vi "LaserPIDPositioning.vi"() -> ()   [LabVIEW 2014]
uses:
  <vilib>/addons/control/pid/pid.llb/PID (DBL).vi
  <vilib>/vision/NI_Vision_Development_Module.lvlib
  <vilib>/addons/control/pid/NI_PID_pid.lvlib
panel:
  out "error out":errorcluster
  in  "error in":errorcluster
  in  "Destination Point":cluster{"DestinationX":dbl, "DestinationY":dbl}
  in  "Horizontal Edge":T1 {"Point2 (Real-World)"."Y" format="%.2f"; "Point2 (Real-World)"."X" format="%.2f"; "Point1 (Real-World)"."Y" format="%.2f"; "Point1 (Real-World)"."X" format="%.2f"; "Point2 (Pixels)"."Y" format="%.2f"; "Point2 (Pixels)"."X" format="%.2f"; "Point1 (Pixels)"."Y" format="%.2f"; "Point1 (Pixels)"."X" format="%.2f"}
  in  "Vertical Edge":T1 {"Point2 (Real-World)"."Y" format="%.2f"; "Point2 (Real-World)"."X" format="%.2f"; "Point1 (Real-World)"."Y" format="%.2f"; "Point1 (Real-World)"."X" format="%.2f"; "Point2 (Pixels)"."Y" format="%.2f"; "Point2 (Pixels)"."X" format="%.2f"; "Point1 (Pixels)"."Y" format="%.2f"; "Point1 (Pixels)"."X" format="%.2f"}
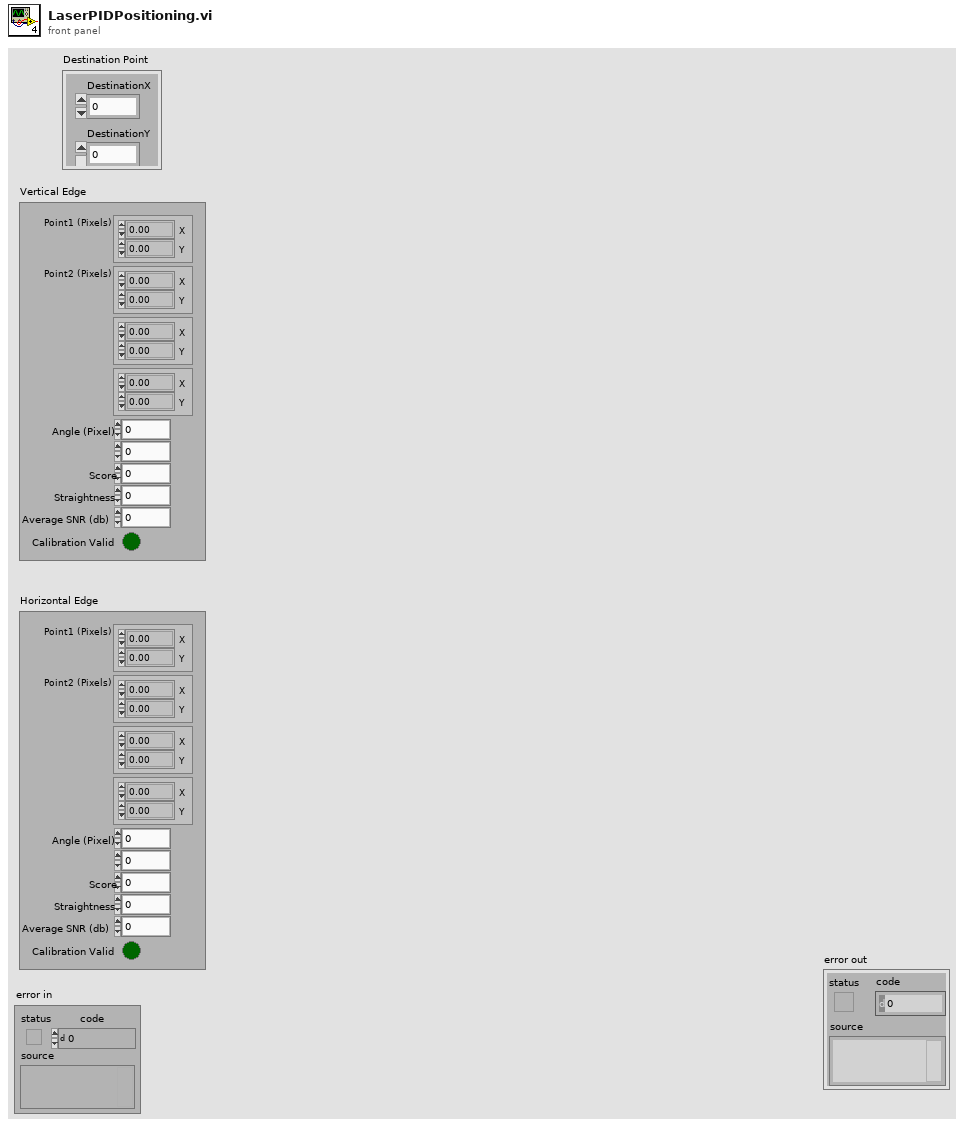
[diagram p1: front panel]
types:
  T1 = cluster{"Point1 (Pixels)":cluster{"X":sgl, "Y":sgl}, "Point2 (Pixels)":cluster{"X":sgl, "Y":sgl}, "Point1 (Real-World)":cluster{"X":sgl, "Y":sgl}, "Point2 (Real-World)":cluster{"X":sgl, "Y":sgl}, "Angle (Pixel)":dbl, "Angle (Real-World)":dbl, "Score":dbl, "Straightness":dbl, "Average SNR (db)":dbl, "Calibration Valid":bool}
  T2 = cluster{"proportional gain (Kc)":dbl, "integral time (Ti, min)":dbl, "derivative time (Td, min)":dbl}
  T3 = cluster{cluster{"X":sgl, "Y":sgl}, cluster{"X":sgl, "Y":sgl}}
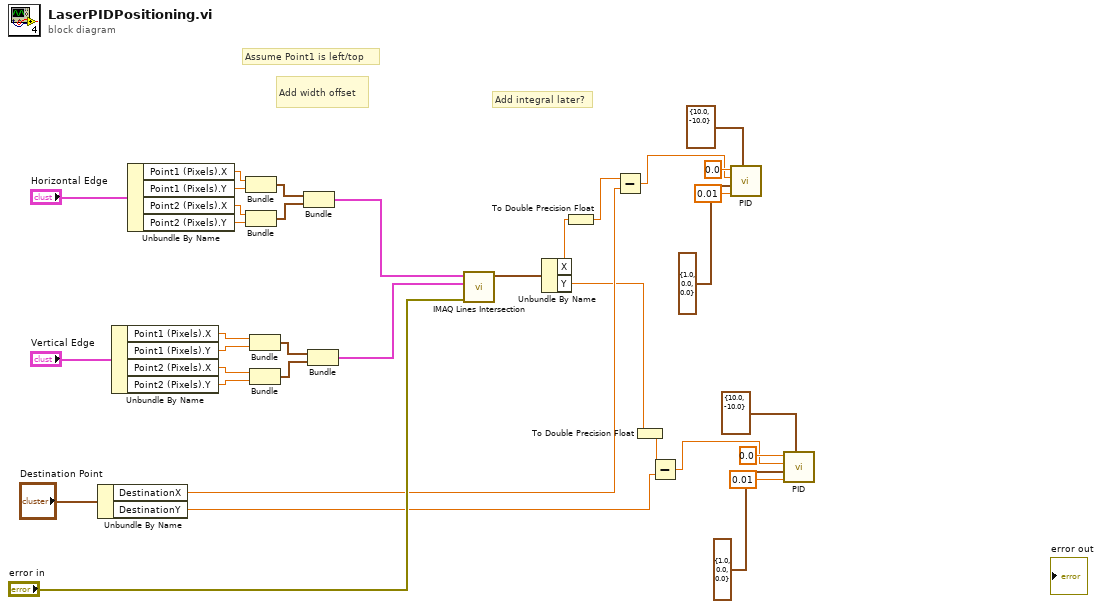
[diagram p0: block diagram]
diagram:
  # "Add integral later?"
  # "Add width offset"
  # "Assume Point1 is left/top"
  n1 = Unbundle By Name("Destination Point") -> ("DestinationX"=w13:dbl, "DestinationY"=w6:dbl)
  n2 = Unbundle By Name("Vertical Edge") -> ("Point1 (Pixels).X"=w23:sgl, "Point1 (Pixels).Y"=w22:sgl, "Point2 (Pixels).X"=w21:sgl, "Point2 (Pixels).Y"=w20:sgl)
  n3 = Unbundle By Name("Horizontal Edge") -> ("Point1 (Pixels).X"=w32:sgl, "Point1 (Pixels).Y"=w31:sgl, "Point2 (Pixels).X"=w30:sgl, "Point2 (Pixels).Y"=w29:sgl)
  n4 = Bundle("X"=w32, "Y"=w31) -> (w28:cluster{"X":sgl, "Y":sgl})  [unwired: 1 in]
  n5 = Bundle("X"=w30, "Y"=w29) -> (w27:cluster{"X":sgl, "Y":sgl})  [unwired: 1 in]
  n6 = Bundle("X"=w23, "Y"=w22) -> (w25:cluster{"X":sgl, "Y":sgl})  [unwired: 1 in]
  n7 = Bundle("X"=w21, "Y"=w20) -> (w24:cluster{"X":sgl, "Y":sgl})  [unwired: 1 in]
  n8 = Bundle(w28, w27) -> (w26:T3)  [unwired: 1 in]
  n9 = Bundle(w25, w24) -> (w19:T3)  [unwired: 1 in]
  n10 = call "IMAQ Lines Intersection"("error in (no error)"="error in", "Line 2"=w19, "Line 1"=w26) -> ("Intersection Point"=w17:cluster{"X":sgl, "Y":sgl})  [unwired: 6 in, 2 out]
  n11 = Unbundle By Name(w17) -> ("X"=w3:sgl, "Y"=w7:sgl)
  n12 = To Double Precision Float(number=w3) -> (double precision float=w2:dbl)
  n13 = Subtract(x=w2, y=w13) -> (x-y=w12:dbl)
  n14 = To Double Precision Float(number=w7) -> (double precision float=w1:dbl)
  n15 = Subtract(x=w1, y=w6) -> (x-y=w8:dbl)
  n16 = call-poly <vilib>:"PID.vi"("output range"=cluster{"output high":dbl, "output low":dbl} {"output high"=10.0, "output low"=-10.0}, "dt (s)"=0.01, "PID gains"=T2 {"proportional gain (Kc)"=1.0, "integral time (Ti, min)"=0.0, "derivative time (Td, min)"=0.0}, "process variable"=w12, "setpoint"=0.0) -> ()  [unwired: 5 in, 2 out]
  n17 = call-poly <vilib>:"PID.vi"("output range"=cluster{"output high":dbl, "output low":dbl} {"output high"=10.0, "output low"=-10.0}, "dt (s)"=0.01, "PID gains"=T2 {"proportional gain (Kc)"=1.0, "integral time (Ti, min)"=0.0, "derivative time (Td, min)"=0.0}, "process variable"=w8, "setpoint"=0.0) -> ()  [unwired: 5 in, 2 out]
